vi "Percent-Encode Query.vi"(10 "Query":string) -> (2 "Pct-Encoded Query":string)   [LabVIEW 2013, in "openURI.lvlib" / "URI-Component.Query.lvclass"]
uses:
  URI-Component.Query.lvclass
  openURI.lvlib
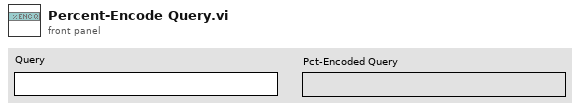
[diagram p1: front panel]
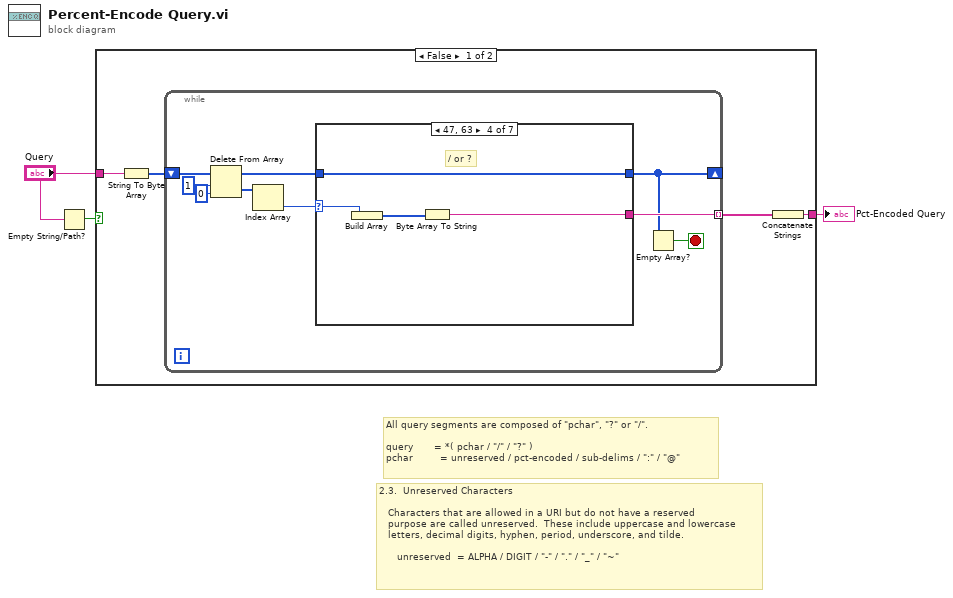
[diagram p0: block diagram]
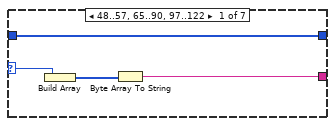
[diagram p2: hidden frame]
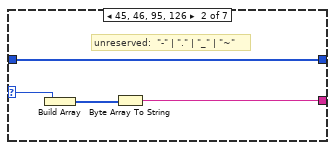
[diagram p3: hidden frame]
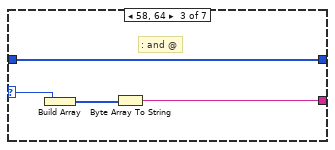
[diagram p4: hidden frame]
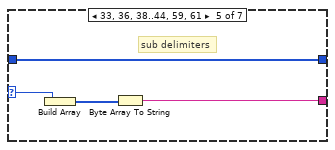
[diagram p5: hidden frame]
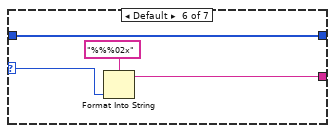
[diagram p6: hidden frame]
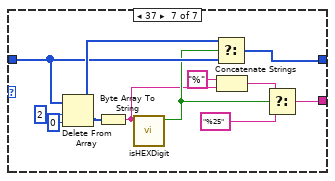
[diagram p7: hidden frame]
diagram:
  # "2.3.  Unreserved Characters\n\n   Characters that are allowed in a URI but do not have a reserved\n   purpose are called unreserved.  These include uppercase and lowercase\n   letters, decimal digits, hyphen, period, underscore, and tilde.\n\n      unreserved  = ALPHA / DIGIT / \"-\" / \".\" / \"_\" / \"~\""
  # "All query segments are composed of \"pchar\", \"?\" or \"/\".\n\nquery       = *( pchar / \"/\" / \"?\" )\npchar         = unreserved / pct-encoded / sub-delims / \":\" / \"@\""
  n1 = Empty String/Path?(string/path="Query") -> (empty?=w2:bool)
  n2 = case shown="False" w2 {
    tunnel: "Query" -> [w5 _]
    tunnel: [w4 _] -> w3
    frame False {
      n3 = String To Byte Array(string=w5) -> (unsigned byte array=w7:u8[])
      n4 = while {
        tunnel: [w16] -> w6 mode=indexing
        shift-right: [w9] -> _
        shift-left: w7 -> [w15]
        stop <- w8 stop-if-true
        n5 = Delete From Array(array=w15, length=1, index=0) -> (deleted portion=w12:u8[], array with subset deleted=w10:u8[])
        n6 = Index Array(array=w12) -> (element=w11:u8)  [unwired: 1 in]
        n7 = case shown="47, 63" w11 {
          selector: w11 -> [w20 w24 w28 w32 w36 w40 _]
          tunnel: [w18 w22 w26 w30 w34 w38 w45] -> w16
          tunnel: w10 -> [w17 w21 w25 w29 w33 w37 w48]
          tunnel: [w17 w21 w25 w29 w33 w37 w47] -> w9
          frame 48..57, 65..90, 97..122 {
            n8 = Build Array(w20) -> (w19:u8[])
            n9 = Byte Array To String(unsigned byte array=w19) -> (string=w18:string)
          }
          frame 45, 46, 95, 126 {
            # "unreserved:  \"-\" | \".\" | \"_\" | \"~\""
            n10 = Build Array(w24) -> (w23:u8[])
            n11 = Byte Array To String(unsigned byte array=w23) -> (string=w22:string)
          }
          frame 58, 64 {
            # ": and @"
            n12 = Build Array(w28) -> (w27:u8[])
            n13 = Byte Array To String(unsigned byte array=w27) -> (string=w26:string)
          }
          frame 47, 63 {
            # "/ or ?"
            n14 = Build Array(w32) -> (w31:u8[])
            n15 = Byte Array To String(unsigned byte array=w31) -> (string=w30:string)
          }
          frame 33, 36, 38..44, 59, 61 {
            # "sub delimiters"
            n16 = Build Array(w36) -> (w35:u8[])
            n17 = Byte Array To String(unsigned byte array=w35) -> (string=w34:string)
          }
          frame Default {
            n18 = Format Into String(format string="%%%02x", w40) -> (resulting string=w38:string)  [unwired: 2 in, 1 out]
          }
          frame 37 {
            n19 = Delete From Array(array=w48, length=2, index=0) -> (deleted portion=w50:u8[], array with subset deleted=w49:u8[])
            n20 = Byte Array To String(unsigned byte array=w50) -> (string=w43:string)
            n21 = call "isHEXDigit.vi"("characters"=w43) -> ("HEX Digits"=w46:bool)  [unwired: 10 in]
            n22 = Select(t=w49, s=w46, f=w48) -> (s? t:f=w47:u8[])
            n23 = Concatenate Strings("%" ("string"), w43) -> (w42:string)
            n24 = Select(t=w42, s=w46, f="%25" ("string")) -> (s? t:f=w45:string)
          }
        }
        n25 = Empty Array?(array=w9) -> (empty?=w8:bool)
      }
      n26 = Concatenate Strings(w6) -> (w4:string)
    }
    frame True {
    }
  }
  "Pct-Encoded Query" <- w3
